vi "add_scan_data.vi"(8 "error in (no error)":errorcluster, 10 "single scan data":string[](array[string]), 11 "Analysis in":refnum<class "Analysis.lvclass">) -> (0 "error out":errorcluster, 3 "Analysis out":refnum<class "Analysis.lvclass">)   [LabVIEW 2017, in "Analysis.lvclass"]
doc: "adds data to the scan data arrray (isotope_name, magnet_value, signal).\nThe full array is 3-dim array in order to store multiple sets of data (e.g. scans for each isotope).\n\nInput is a 1-dim array that holds one single point of a scan (isotope_name, magnet_value, signal)"
uses:
  Analysis.lvclass
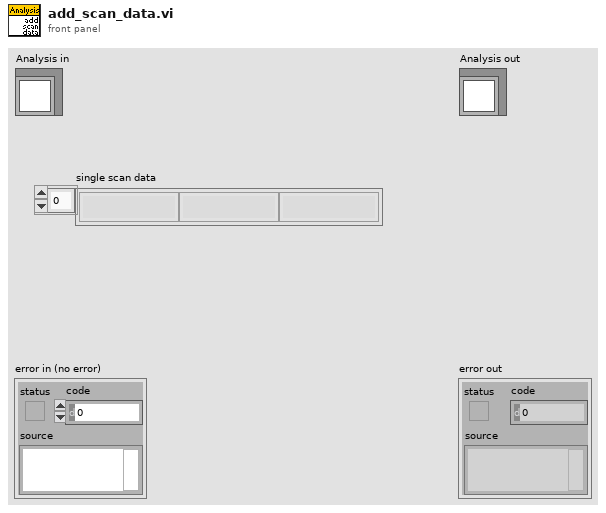
[diagram p1: front panel]
types:
  T1 = typedef "ScanDataArray_new.ctl" = cluster{"scan data":string[][]}[]
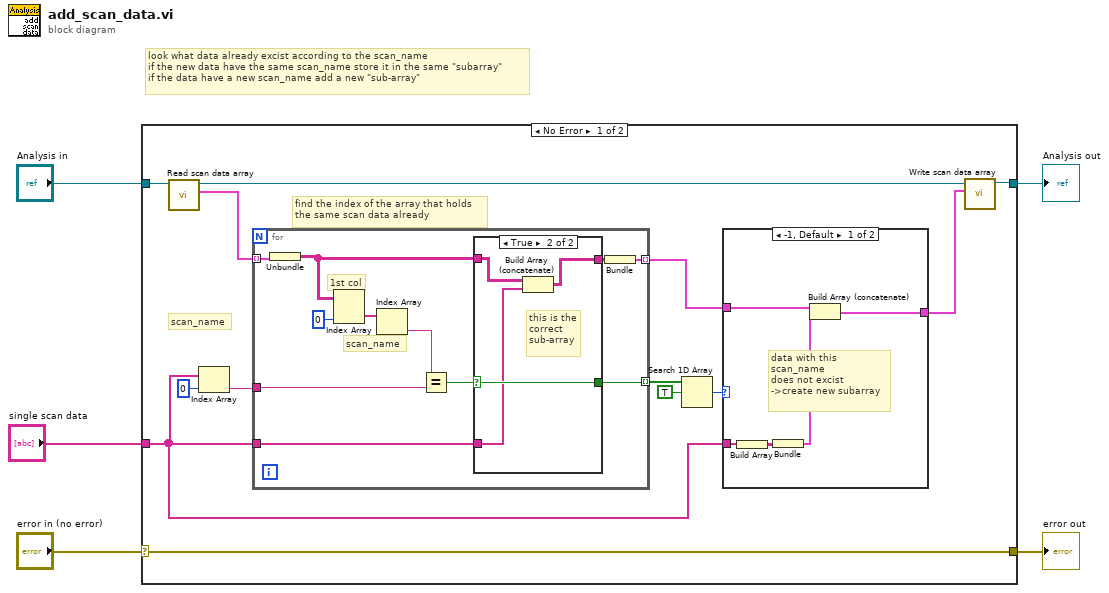
[diagram p0: block diagram]
diagram:
  # "look what data already excist according to the scan_name\nif the new data have the same scan_name store it in the same \"subarray\"\nif the data have a new scan_name add a new \"sub-array\""
  n1 = case shown="No Error" "error in (no error)" {
    selector: "error in (no error)" -> [w18 w43]
    tunnel: [w18 w43] -> w4
    tunnel: [w15 w42] -> w2
    tunnel: "Analysis in" -> [w17 w42]
    tunnel: "single scan data" -> [w6 _]
    frame No Error {
      # "find the index of the array that holds\nthe same scan data already"
      # "scan_name"
      n2 = call-dynamic "Read scan data array.vi"("Analysis in"=w17) -> ("scan data array"=w13:T1, "Analysis out"=w16:refnum<class "Analysis.lvclass">)  [unwired: 8 in, 1 out]
      n3 = Index Array(array=w6, index=0) -> (element=w11:string)
      n4 = for {
        tunnel: w13 -> [w28] mode=indexing
        tunnel: w11 -> [w32]
        tunnel: [w29] -> w12 mode=indexing
        tunnel: [w26] -> w8 mode=indexing
        tunnel: w6 -> [w31]
        # "scan_name"
        # "1st col"
        n5 = Unbundle(w28) -> ("scan data"=w27:string[][])
        n6 = Index Array(array=w27, index (col)=0 ("disabled index (col)")) -> (element=w34:string[])  [unwired: 1 in]
        n7 = Index Array(array=w34) -> (element=w33:string)  [unwired: 1 in]
        n8 = Equal?(x=w33, y=w32) -> (x = y?=w30:bool)
        n9 = case shown="True" w30 {
          selector: w30 -> [w37 w41]
          tunnel: w31 -> [_ w38]
          tunnel: [w37 w41] -> w29
          tunnel: w27 -> [w36 w40]
          tunnel: [w36 w39] -> w25
          frame False {
            # "not the right\nsub-array"
          }
          frame True {
            # "this is the\ncorrect\nsub-array"
            n10 = Build Array (concatenate)(w40, w38) -> (w39:string[][])
          }
        }
        n11 = Bundle("scan data"=w25) -> (w26:cluster{"scan data":string[][]})  [unwired: 1 in]
      }
      n12 = Search 1D Array(1D array=w12, element=TRUE) -> (index of element=w9:i32)  [unwired: 1 in]
      n13 = case shown="-1, Default" w9 {
        tunnel: w8 -> [w21 w24]
        tunnel: w6 -> [w23 _]
        tunnel: [w22 w24] -> w7
        frame -1, Default {
          # "data with this\nscan_name\ndoes not excist\n->create new subarray"
          n14 = Build Array(w23) -> (w20:string[][])
          n15 = Bundle(w20) -> (w19:cluster{string[][]})  [unwired: 1 in]
          n16 = Build Array (concatenate)(w21, w19) -> (w22:cluster{"scan data":string[][]}[])
        }
        frame 0.. {
          # "all fine, data have been\ninserted already"
        }
      }
      n17 = call-dynamic "Write scan data array.vi"("scan data array"=w7, "Analysis in"=w16) -> ("Analysis out"=w15:refnum<class "Analysis.lvclass">)  [unwired: 8 in, 1 out]
    }
    frame Error {
    }
  }
  "error out" <- w4
  "Analysis out" <- w2
